vi "13.vi"() -> ()   [LabVIEW 2023]
uses:
  <vilib>/Utility/file.llb/Read Delimited Spreadsheet (DBL).vi
  <vilib>/Utility/file.llb/Write Delimited Spreadsheet (I64).vi
panel:
  in  "citeste":bool
  in  "salveaza":bool
  out "length":i32[][](array[numeric])
  in  "calculeaza":bool
  in  "stop":bool
  in  "Table Control":string[][](table)
  out "Waveform Graph":dbl[][](graph)
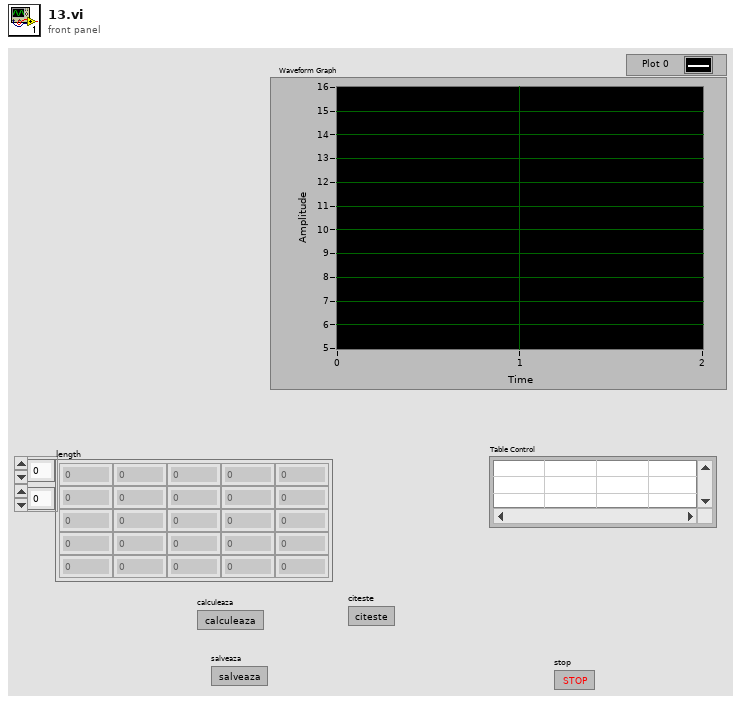
[diagram p1: front panel]
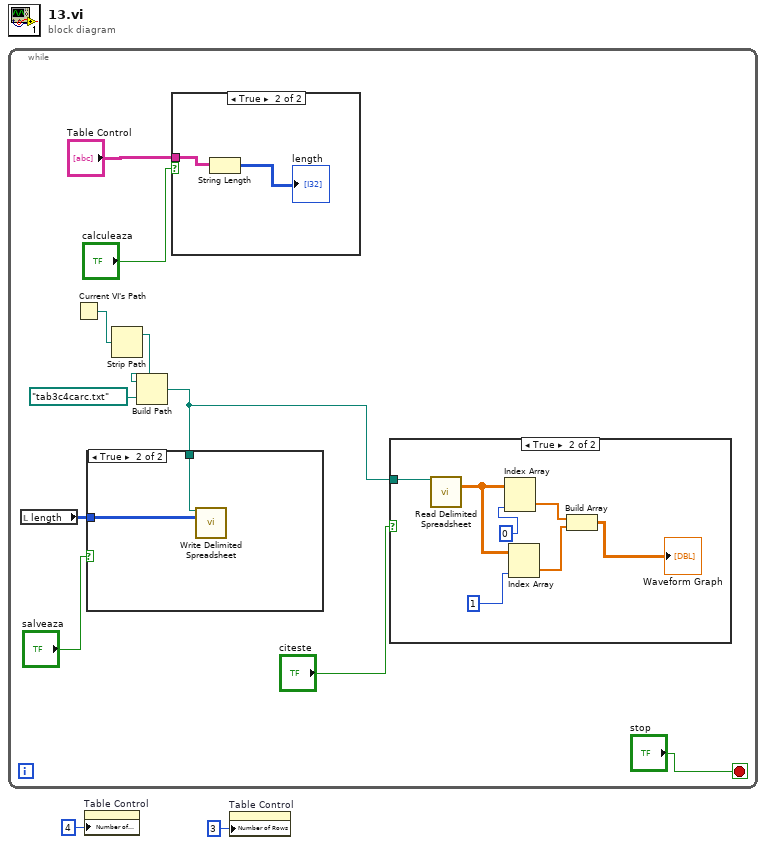
[diagram p0: block diagram]
diagram:
  n1 = while {
    stop <- "stop" stop-if-true
    n2 = local read "length"() -> (w6:i32[][])
    n3 = Current VI's Path() -> (path=w9:path)
    n4 = Strip Path(path=w9) -> (stripped path=w8:path)  [unwired: 1 out]
    n5 = Build Path(base path=w8, name or relative path=path "tab3c4carc.txt") -> (appended path=w4:path)
    n6 = case shown="True" "salveaza" {
      tunnel: w6 -> [_ w21]
      tunnel: w4 -> [_ w20]
      frame False {
      }
      frame True {
        n7 = call-poly <vilib>:"Write Delimited Spreadsheet.vi"("file path (dialog if empty)"=w20, "2D data"=w21) -> ()  [unwired: 12 in, 2 out]
      }
    }
    n8 = case shown="True" "calculeaza" {
      tunnel: "Table Control" -> [_ w23]
      frame False {
      }
      frame True {
        n9 = String Length(string=w23) -> (length=→"length":i32[][])
      }
    }
    n10 = case shown="True" "citeste" {
      tunnel: w4 -> [_ w19]
      frame False {
      }
      frame True {
        n11 = call-poly <vilib>:"Read Delimited Spreadsheet.vi"("file path (dialog if empty)"=w19) -> ("all rows"=w18:dbl[][])  [unwired: 9 in, 5 out]
        n12 = Index Array(array=w18, index (col)=0 ("index (row)")) -> (element=w17:dbl[])  [unwired: 1 in]
        n13 = Index Array(array=w18, index (col)=1 ("index (row)")) -> (element=w16:dbl[])  [unwired: 1 in]
        n14 = Build Array(w17, w16) -> (→"Waveform Graph":dbl[][])
      }
    }
  }
  n15 = property on="Table Control" class="Tbl (strict)"("Number of Columns"=u32 4) -> ()  [unwired: 2 in, 2 out]
  n16 = property on="Table Control" class="Tbl (strict)"("Number of Rows"=u32 3) -> ()  [unwired: 2 in, 2 out]
